vi "Brake.vi"(8 "Brake!":bool, 11 "error in (no error)":errorcluster) -> (3 "error out":errorcluster)   [LabVIEW 2016]
doc: "Inputs\nBrake\n\nOutputs\n-\n\nActivates the brake motor if the boolean input is true. It brakes for 3 seconds and then goes in reverse direction for 1 second to make sure the brake is not activated on the next run."
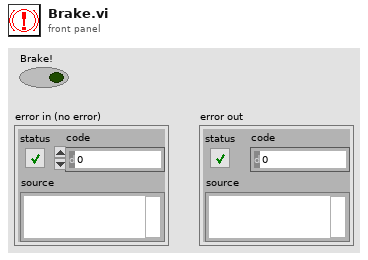
[diagram p1: front panel]
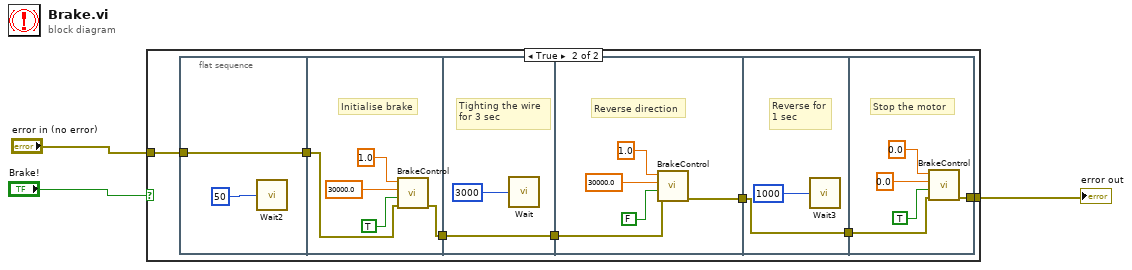
[diagram p0: block diagram]
diagram:
  n1 = case shown="True" "Brake!" {
    tunnel: "error in (no error)" -> [w4 w11]
    tunnel: [w4 w6] -> w3
    frame False {
    }
    frame True {
      n2 = flat-sequence {
        tunnel: w11 -> [w13]
        tunnel: [w13] -> w5
        tunnel: [w14] -> w9
        tunnel: w5 -> [w15]
        tunnel: [w19] -> w10
        tunnel: w9 -> [w19]
        tunnel: [w22] -> w7
        tunnel: w10 -> [w21]
        tunnel: [w26] -> w8
        tunnel: w7 -> [w26]
        tunnel: w8 -> [w28]
        tunnel: [w29] -> w6
        frame #0 {
          n3 = call "Wait2"("Count(mSec)"=u32 50) -> ()  [unwired: 1 out]
        }
        frame #1 {
          # "Initialise brake"
          n4 = call "BrakeControl.vi"("error in (no error)"=w15, "Digital Input"=TRUE, "Frequency [Hz]"=30000.0, "Duty Cycle"=1.0) -> ("error out"=w14:errorcluster)  [unwired: 7 in]
        }
        frame #2 {
          # "Tighting the wire\nfor 3 sec"
          n5 = call "Wait"("Count(mSec)"=u32 3000) -> ()  [unwired: 1 out]
        }
        frame #3 {
          # "Reverse direction"
          n6 = call "BrakeControl.vi"("error in (no error)"=w21, "Digital Input"=FALSE, "Frequency [Hz]"=30000.0, "Duty Cycle"=1.0) -> ("error out"=w22:errorcluster)  [unwired: 7 in]
        }
        frame #4 {
          # "Reverse for\n1 sec"
          n7 = call "Wait3"("Count(mSec)"=u32 1000) -> ()  [unwired: 1 out]
        }
        frame #5 {
          # "Stop the motor"
          n8 = call "BrakeControl.vi"("error in (no error)"=w28, "Digital Input"=TRUE, "Frequency [Hz]"=0.0, "Duty Cycle"=0.0) -> ("error out"=w29:errorcluster)  [unwired: 7 in]
        }
      }
    }
  }
  "error out" <- w3
